vi "条件结构隧道.vi"() -> ()   [LabVIEW 2022 SP3]
doc: "本VI是为《我和LabVIEW》一书编写的示例。\n关于本书的介绍请参考网页：\nhttp://ruanqizhen.spaces.live.com/blog/cns!5852D4F797C53FB6!4310.entry"
panel:
  out "数值输出":dbl
  in  "数值":dbl
  in  "单选按钮":T1(radio)
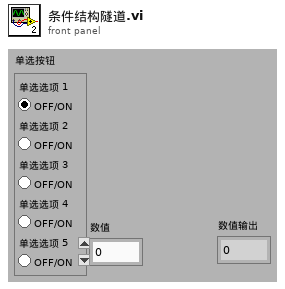
[diagram p1: front panel]
types:
  T1 = enum32{"单选选项 1", "单选选项 2", "单选选项 3", "单选选项 4", "单选选项 5"}
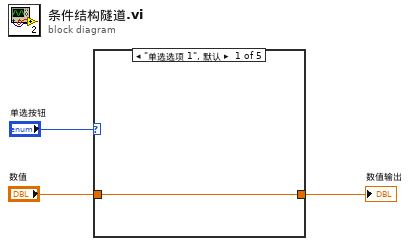
[diagram p0: block diagram]
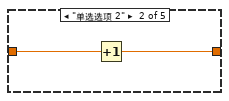
[diagram p2: hidden frame]
diagram:
  n1 = case shown="\"单选选项 1\", 默认" "单选按钮" {
    tunnel: [w4 w5 w7 w8 w9] -> w1
    tunnel: "数值" -> [w4 w6 w7 w8 w9]
    frame "单选选项 1", Default {
    }
    frame "单选选项 2" {
      n2 = Increment(x=w6) -> (x+1=w5:dbl)
    }
    frame "单选选项 3" {
    }
    frame "单选选项 4" {
    }
    frame "单选选项 5" {
    }
  }
  "数值输出" <- w1
